vi "Parse server response.vi"(8 "error in (no error)":errorcluster, 11 "server response in":string) -> (0 "error out":errorcluster, 1 "detailed err description":string, 2 "JSON out":string, 3 "binary data":u8[](array[numeric]), 4 "Protocoll version":u8, 5 "short err code":u8, 6 "optional header":u8[](array[numeric]))   [LabVIEW 2018, in "LV-Julia_ZMQ-Roundtrip_lib.lvlib"]
uses:
  LV-Julia_ZMQ-Roundtrip_lib.lvlib
  <vilib>/Utility/error.llb/Error Cluster From Error Code.vi
  <vilib>/ErrorRing/Error Ring.xnode
panel:
  out "JSON err":string
  out "binary data length":u32
  out "Error JSON length":u32
  out "optional header length":u32
  out "unsigned byte array":u8[](array[numeric])
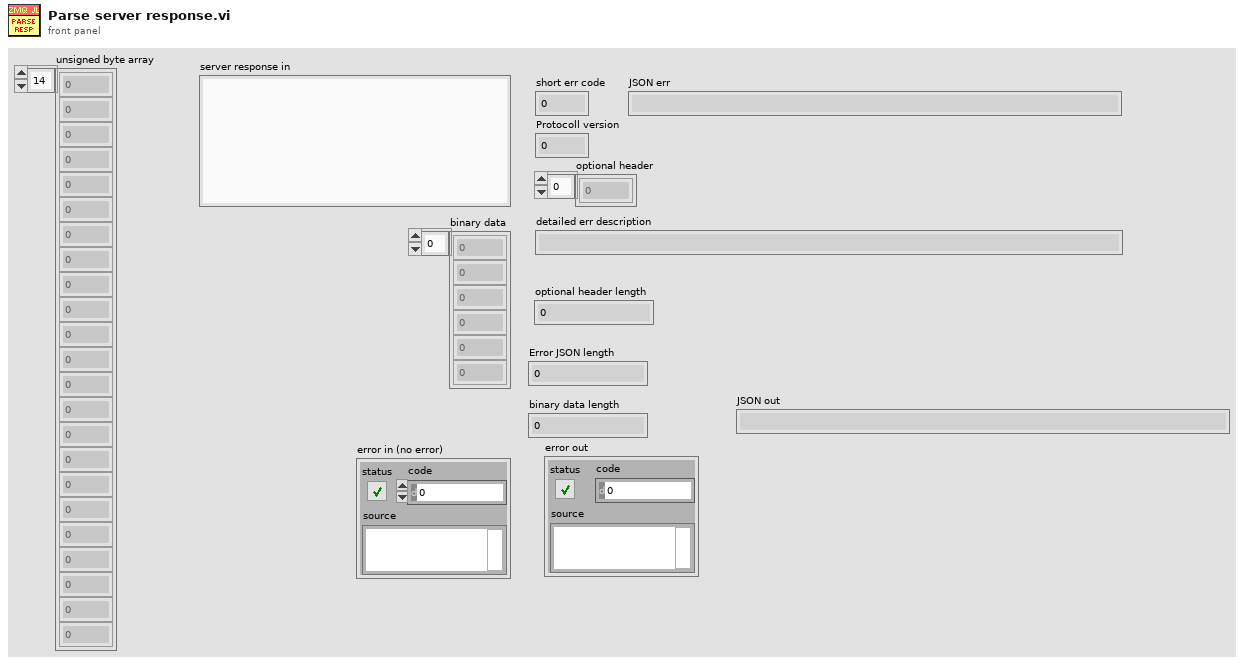
[diagram p1: front panel]
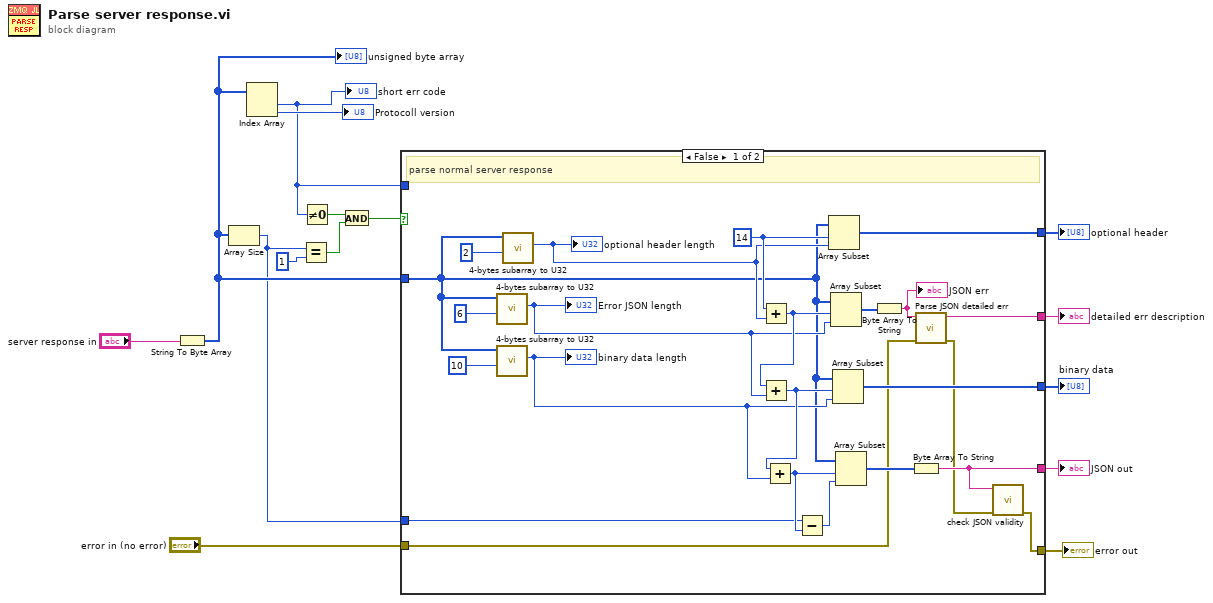
[diagram p0: block diagram]
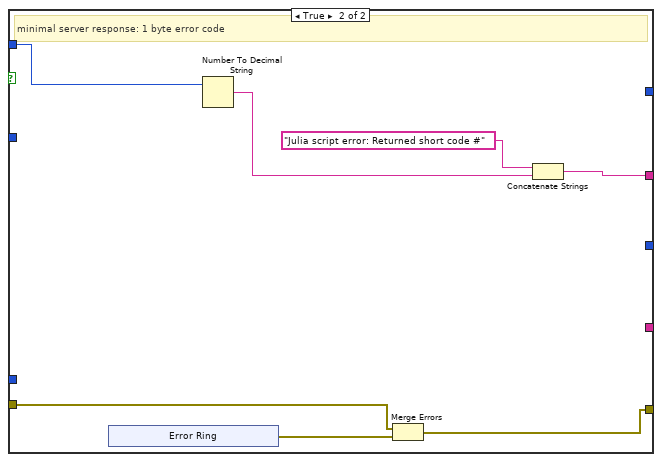
[diagram p2: hidden frame]
diagram:
  n1 = String To Byte Array(string="server response in") -> (unsigned byte array=w7:u8[])
  "unsigned byte array" <- w7
  n2 = Array Size(array=w7) -> (size(s)=w6:i32)
  n3 = Index Array(array=w7) -> (element #1=w1:u8, element #2=→"Protocoll version":u8)  [unwired: 2 in]
  "short err code" <- w1
  n4 = Equal?(x=w6, y=1) -> (x = y?=w3:bool)
  n5 = Not Equal To 0?(x=w1) -> (x != 0?=w4:bool)
  n6 = And(x=w4, y=w3) -> (x .and. y?=w2:bool)
  n7 = case shown="False" w2 {
    tunnel: [w35 _] -> w13
    tunnel: [w30 w40] -> w12
    tunnel: [w27 _] -> w11
    tunnel: w7 -> [w16 _]
    tunnel: "error in (no error)" -> [w21 w43]
    tunnel: [w20 _] -> w9
    tunnel: [w18 w44] -> w8
    tunnel: w6 -> [w17 _]
    tunnel: w1 -> [_ w42]
    frame False {
      w34 = 14 ("index")
      # "parse normal server response"
      n8 = call "4-bytes subarray to U32.vi"("offset"=6 ("index"), "unsigned byte array"=w16) -> ("U32 Out"=w28:u32)  [unwired: 8 in, 1 out]
      "Error JSON length" <- w28
      n9 = call "4-bytes subarray to U32.vi"("offset"=10 ("index"), "unsigned byte array"=w16) -> ("U32 Out"=w25:u32)  [unwired: 8 in, 1 out]
      "binary data length" <- w25
      n10 = call "4-bytes subarray to U32.vi"("offset"=2 ("index"), "unsigned byte array"=w16) -> ("U32 Out"=w32:u32)  [unwired: 8 in, 1 out]
      "optional header length" <- w32
      n11 = Add(x=w34, y=w32) -> (x+y=w29:u32)
      n12 = Add(x=w29, y=w28) -> (x+y=w26:u32)
      n13 = Add(x=w26, y=w25) -> (x+y=w24:u32)
      n14 = Subtract(x=w17, y=w24) -> (x-y=w23:u32)
      n15 = Array Subset(array=w16, index=w34, length=w32) -> (w35:u8[])
      n16 = Array Subset(array=w16, index=w29, length=w28) -> (w33:u8[])
      n17 = Array Subset(array=w16, index=w26, length=w25) -> (w27:u8[])
      n18 = Array Subset(array=w16, index=w24, length=w23) -> (w22:u8[])
      n19 = Byte Array To String(unsigned byte array=w33) -> (string=w31:string)
      "JSON err" <- w31
      n20 = Byte Array To String(unsigned byte array=w22) -> (string=w20:string)
      n21 = call "Parse JSON detailed err.vi"("error in (no error)"=w21, "JSON string in"=w31) -> ("error out"=w19:errorcluster, "long err description out"=w30:string)  [unwired: 8 in]
      n22 = call "check JSON validity.vi"("error in (no error)"=w19, "JSON string in"=w20) -> ("error out"=w18:errorcluster)  [unwired: 8 in, 1 out]
    }
    frame True {
      # "minimal server response: 1 byte error code"
      n23 = xnode "Error Ring"() -> ("error out"=w45:errorcluster)
      n24 = Number To Decimal String(number=w42) -> (decimal integer string=w41:string)  [unwired: 1 in]
      n25 = Merge Errors(w43, w45) -> (w44:errorcluster)
      n26 = Concatenate Strings("Julia script error: Returned short code #" ("string"), w41) -> (w40:string)
    }
  }
  "optional header" <- w13
  "error out" <- w8
  "detailed err description" <- w12
  "binary data" <- w11
  "JSON out" <- w9
